vi "NXTMMX-DM.vi"(0 "Input of Motor Multiplexer":T4={"NXTMMX Address"=6, "Which Motor"=0, "Operation"=0, "Next Action"=0, "Position"=0, "Direction"=FALSE, "Power"=100, "Durartion"=0, "Wait for Completion"=FALSE, "Relative"=FALSE} {"Next Action" items=["Float", "Brake"]; "Operation" items=["Run Unlimited", "Run Seconds", "Run Tachometer"]; "Which Motor" items=["Motor 1", "Motor 2", "Both Motors"]; "NXTMMX Address" min=2 max=254 step=2 format="%x"}, 2 "NXT":T2={"error"={"status"=FALSE, "code"=0, "source"=""}, "address"="", "NXT #"=-1, "Show Error"=TRUE, "Connection"=4} {"Connection" items=["USB", "Bluetooth", "USB then Bluetooth", "Last Connection", "Preference"]}, 3 "Input Port":T3 items=["Port 1", "Port 2", "Port 3", "Port 4"]) -> (1 "Output of Motor Multiplexer":T1, 4 "NXT dup":T2={"error"={"status"=FALSE, "code"=0, "source"=""}, "address"="", "NXT #"=-1, "Show Error"=TRUE, "Connection"=4} {"Connection" items=["USB", "Bluetooth", "USB then Bluetooth", "Last Connection", "Preference"]})   [LabVIEW 2009]
uses:
  <vilib>/NXT/Block Support/NXT_InputPort.ctl
  <vilib>/NXT/Subs/LVHSConnector.ctl
  <vilib>/NXT/Block Support/HWPage.SensorType.ctl
  <vilib>/NXT/Block Support/HWPage.SensorMode.ctl
  <vilib>/NXT/Dual Mode Library/Waits/Wait_Num(msec).vi
panel:
  out "Address":i32
  # "mindsensors.com\nCopyright (c) 2009 by mindsensors.com\nEmail: info (<at>) mindsensors (<dot>) com\n\nThis program is free software. You can redistribute it and/or modify\nit under the terms of the GNU General Public License as published by\nthe Free Software Foundation; version 3 of the License.\nRead the license at: http://www.gnu.org/licenses/gpl.txt"
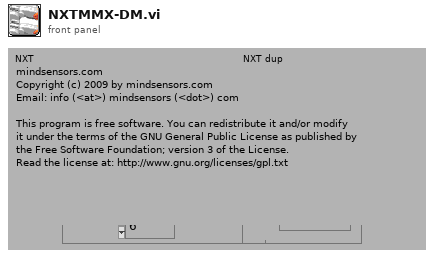
[diagram p1: front panel]
types:
  T1 = cluster{"Milivolts":u16, "Position 1":i32, "Position 2":i32, "Motor battery Voltage":dbl}
  T2 = typedef "LVHSConnector.ctl" = cluster{"error":errorcluster, "address":string, "NXT #":i32, "Show Error":bool, "Connection":u16}
  T3 = typedef "NXT_InputPort.ctl" = u8
  T4 = cluster{"NXTMMX Address":u8, "Which Motor":u8, "Operation":u8, "Next Action":u8, "Position":i32, "Direction":bool, "Power":i8, "Durartion":u8, "Wait for Completion":bool, "Relative":bool}
  T5 = typedef "HWPage.SensorType.ctl" = u8
  T6 = typedef "HWPage.SensorMode.ctl" = u8
  T7 = cluster{"millivolts":i16, "(hi.lo)":u16, "(hi.lo)":u16, dbl}
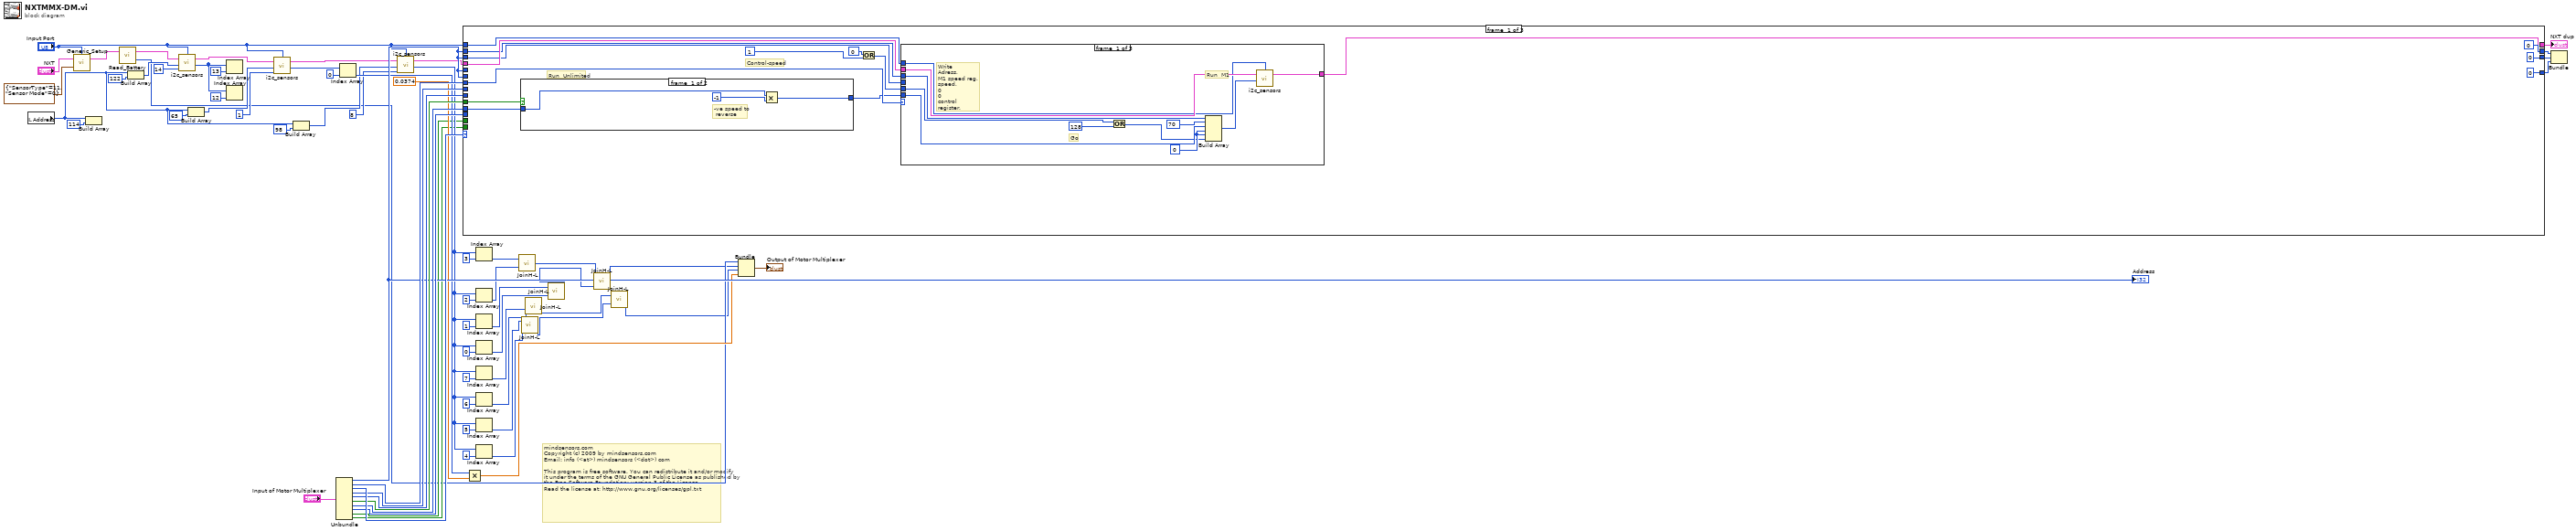
[diagram p0: block diagram]
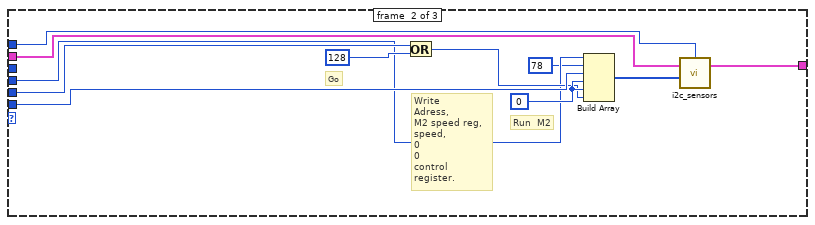
[diagram p2: hidden frame]
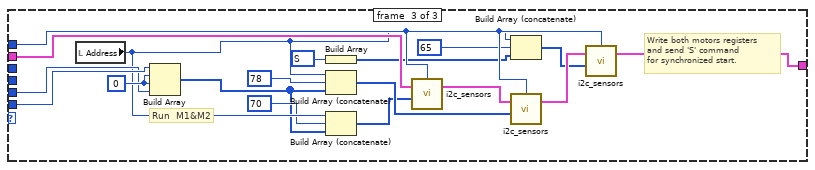
[diagram p3: hidden frame]
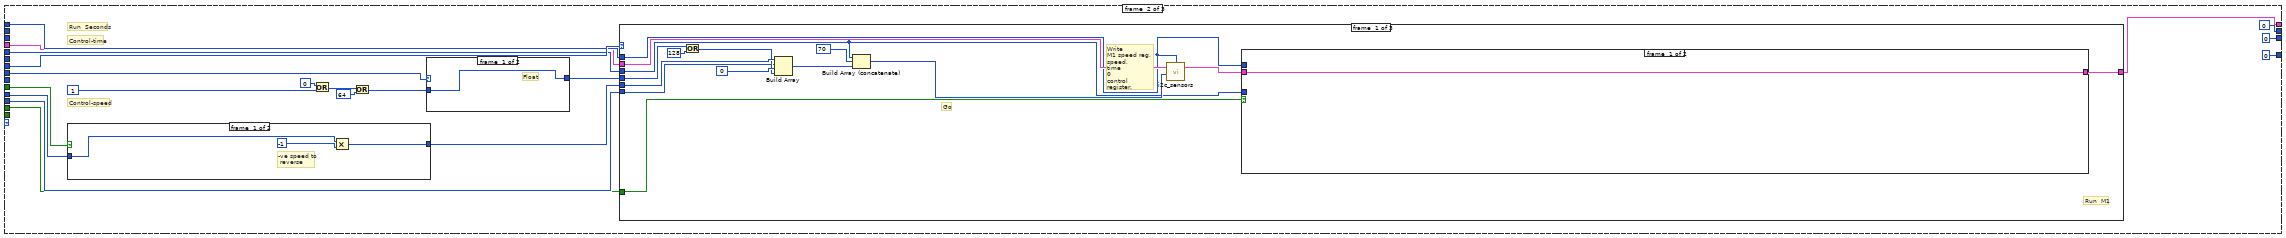
[diagram p5: hidden frame]
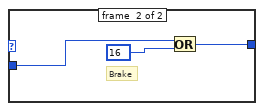
[diagram p6: hidden frame]
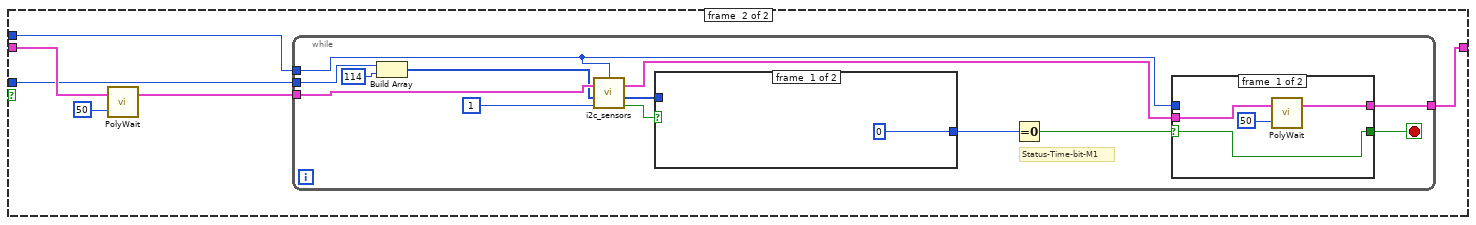
[diagram p7: hidden frame]
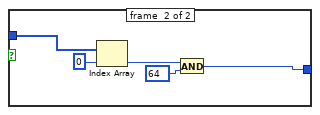
[diagram p9: hidden frame]
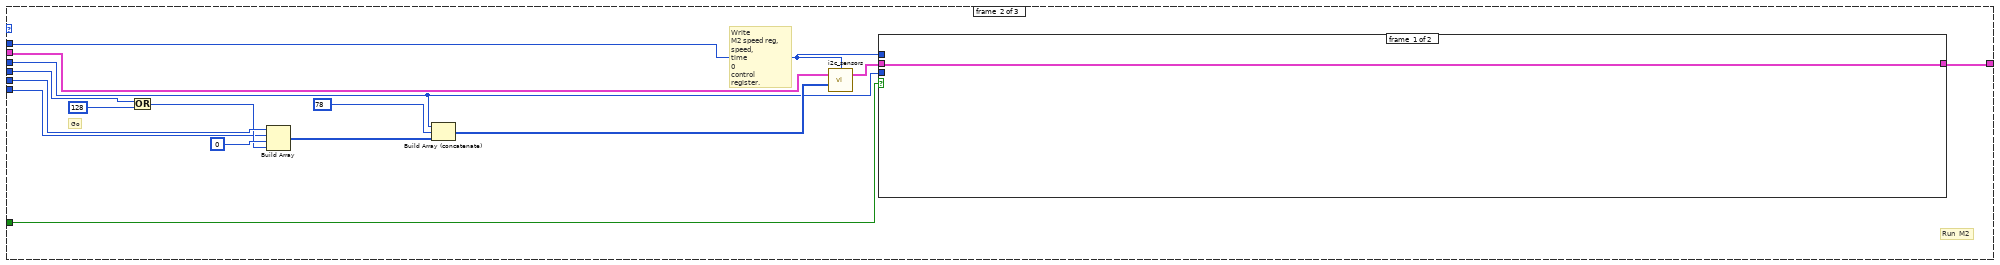
[diagram p10: hidden frame]
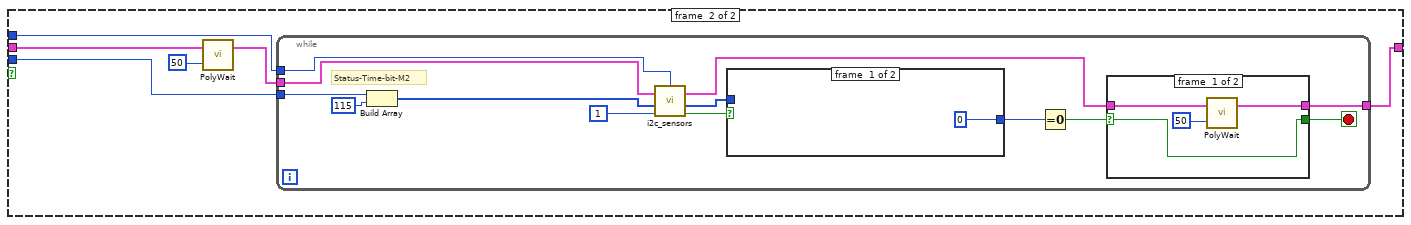
[diagram p11: hidden frame]
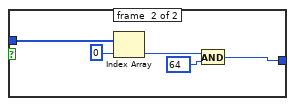
[diagram p13: hidden frame]
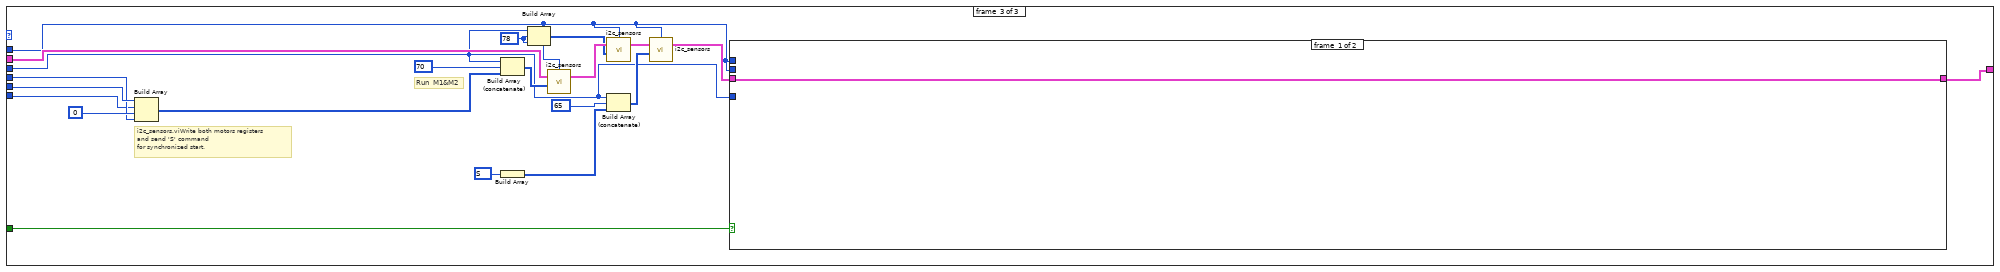
[diagram p14: hidden frame]
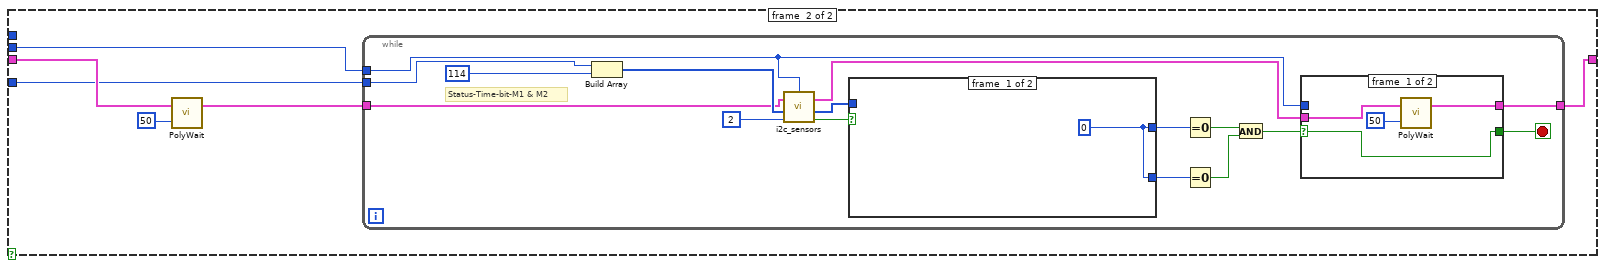
[diagram p15: hidden frame]
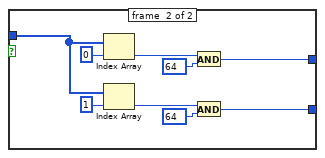
[diagram p17: hidden frame]
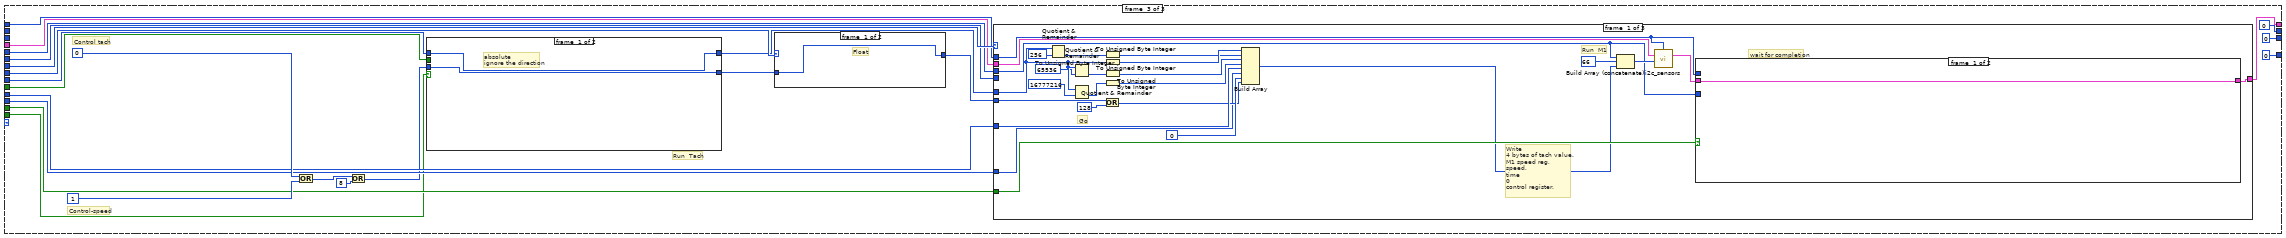
[diagram p19: hidden frame]
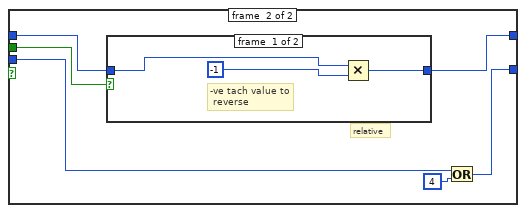
[diagram p20: hidden frame]
diagram:
  # "mindsensors.com\nCopyright (c) 2009 by mindsensors.com\nEmail: info (<at>) mindsensors (<dot>) com\n\nThis program is free software. You can redistribute it and/or modify\nit under the terms of the GNU General Public License as published by\nthe Free Software Foundation; version 3 of the License.\nRead the license at: http://www.gnu.org/licenses/gpl.txt"
  n1 = local read "Address"() -> (w25:i32)
  n2 = call <vilib>:"Generic_Setup.vi"("Sensor Setup"=cluster{"SensorType":T5, "Sensor Mode":T6} {"SensorType"=11, "Sensor Mode"=0}, "NXT"="NXT", "Port"="Input Port") -> ("NXT"=w57:T2)  [unwired: 1 out]
  n3 = Build Array(w25, u8 114 ("Reg Address")) -> ()  [unwired: 1 out]
  n4 = call <vilib>:"Read_Battery.vi"("NXT"=w57) -> ("millivolts"=w20:i16, "NXT"=w28:T2)  [unwired: 2 in]
  n5 = Build Array(w25, u8 122 ("Reg Address")) -> (w42:i32[])
  n6 = call <vilib>:"i2c_sensors.vi"("Return Length"=u8 14 ("bytes to read"), "Bytes to Write"=w42, "NXT"=w28, "Port"="Input Port") -> ("Bytes read"=w40:u8[], "NXT"=w35:T2)  [unwired: 1 in, 1 out]
  n7 = Build Array(w25, u8 65 ("Reg Address")) -> (w37:i32[])
  n8 = Index Array(array=w40, index=13) -> ()  [unwired: 1 out]
  n9 = Index Array(array=w40, index=12) -> ()  [unwired: 1 out]
  n10 = call <vilib>:"i2c_sensors.vi"("Return Length"=u8 1 ("bytes to read"), "Bytes to Write"=w37, "NXT"=w35, "Port"="Input Port") -> ("Bytes read"=w36:u8[], "NXT"=w30:T2)  [unwired: 1 in, 1 out]
  n11 = Build Array(w25, u8 98 ("Reg Address")) -> (w34:i32[])
  n12 = Unbundle("Input of Motor Multiplexer") -> ("NXTMMX Address"=w59:u8, "Which Motor"=w61:u8, "Operation"=w66:u8, "Next Action"=w65:u8, "Position"=w63:i32, "Direction"=w62:bool, "Power"=w64:i8, "Durartion"=w60:u8, "Wait for Completion"=w22:bool, "Relative"=w21:bool)
  "Address" <- w59
  n13 = Index Array(array=w36, index=0) -> (element=w45:u8)
  n14 = call <vilib>:"i2c_sensors.vi"("Return Length"=u8 8 ("bytes to read"), "Bytes to Write"=w34, "NXT"=w30, "Port"="Input Port") -> ("Bytes read"=w31:u8[], "NXT"=w26:T2)  [unwired: 1 in, 1 out]
  n15 = case shown="2" w66 {
    tunnel: w62 -> [w80 w144 w330]
    tunnel: w64 -> [w79 w143 w320]
    tunnel: w61 -> [w78 w142 w329]
    tunnel: "Input Port" -> [w76 w140 w328]
    tunnel: w60 -> [_ w137 w325]
    tunnel: w65 -> [_ w136 w324]
    tunnel: w63 -> [_ _ w321]
    tunnel: w22 -> [_ w133 w322]
    tunnel: w21 -> [_ _ w318]
    tunnel: [0 0 0] -> w19
    tunnel: [u32 0 ("Out") u32 0 ("Out") u32 0 ("Out")] -> w18
    tunnel: [u16 0 u16 0 u16 0] -> w17
    tunnel: w26 -> [w71 w129 w311]
    tunnel: [w70 w128 w312] -> w16
    tunnel: w59 -> [_ w127 w310]
    tunnel: w59 -> [w69 _ _]
    tunnel: w59 -> [_ _ w309]
    tunnel: w59 -> [w68 _ _]
    frame #0 {
      # "Control-speed"
      # "Run  Unlimited"
      n16 = case shown="False" w80 {
        tunnel: w79 -> [w125 w126]
        tunnel: [w123 w126] -> w77
        frame #0 {
          # "-ve speed to\n reverse"
          n17 = Multiply(x=w125, y=i8 -1) -> (x*y=w123:i8)
        }
        frame #1 {
        }
      }
      n18 = Or(x=0, y=1) -> (x .or. y?=w75:i32)
      n19 = case shown="2" w78 {
        tunnel: w75 -> [w92 w103 w119]
        tunnel: w77 -> [w91 w102 w122]
        tunnel: w76 -> [w86 w99 w114]
        tunnel: w71 -> [w88 w98 w118]
        tunnel: [w87 w97 w109] -> w70
        tunnel: w69 -> [w85 _ _]
        tunnel: w68 -> [_ w96 _]
        frame #0 {
          w90 = 0
          # "Go"
          # "Run  M1"
          # "Write \nAdress,\nM1 speed reg,\nspeed,\n0\n0\ncontrol register."
          n20 = Or(x=w92, y=128) -> (x .or. y?=w89:i32)
          n21 = Build Array(w85, 70, w91, w90, w90, w89) -> (w83:i32[])
          n22 = call <vilib>:"i2c_sensors.vi"("Bytes to Write"=w83, "NXT"=w88, "Port"=w86) -> ("NXT"=w87:T2)  [unwired: 2 in, 2 out]
        }
        frame #1 {
          w101 = 0
          # "Go"
          # "Run  M2"
          # "Write\nAdress, \nM2 speed reg,\nspeed,\n0\n0\ncontrol register."
          n23 = Or(x=w103, y=128) -> (x .or. y?=w100:i32)
          n24 = Build Array(w96, 78, w102, w101, w101, w100) -> (w94:i32[])
          n25 = call <vilib>:"i2c_sensors.vi"("Bytes to Write"=w94, "NXT"=w98, "Port"=w99) -> ("NXT"=w97:T2)  [unwired: 2 in, 2 out]
        }
        frame #2 {
          w120 = u16 83 items=["S"=83]
          w121 = 0
          # "Write both motors registers\nand send 'S' command \nfor synchronized start."
          # "Run  M1&M2"
          n26 = local read "Address"() -> (w108:i32)
          n27 = Build Array(w122, w121, w121, w119) -> (w105:i32[])
          n28 = Build Array(w120) -> (w112:u16[])
          n29 = Build Array (concatenate)(w108, 78, w105) -> (w116:i32[])
          n30 = Build Array (concatenate)(w108, 70, w105) -> (w106:i32[])
          n31 = call <vilib>:"i2c_sensors.vi"("Bytes to Write"=w106, "NXT"=w118, "Port"=w114) -> ("NXT"=w115:T2)  [unwired: 2 in, 2 out]
          n32 = Build Array (concatenate)(w108, 65, w112) -> (w110:i32[])
          n33 = call <vilib>:"i2c_sensors.vi"("Bytes to Write"=w116, "NXT"=w115, "Port"=w114) -> ("NXT"=w113:T2)  [unwired: 2 in, 2 out]
          n34 = call <vilib>:"i2c_sensors.vi"("Bytes to Write"=w110, "NXT"=w113, "Port"=w114) -> ("NXT"=w109:T2)  [unwired: 2 in, 2 out]
        }
      }
    }
    frame #1 {
      # "Control-time"
      # "Control-speed"
      # "Run  Seconds"
      n35 = case shown="False" w144 {
        tunnel: w143 -> [w307 w308]
        tunnel: [w305 w308] -> w141
        frame #0 {
          # "-ve speed to\n reverse"
          n36 = Multiply(x=w307, y=i8 -1) -> (x*y=w305:i8)
        }
        frame #1 {
        }
      }
      n37 = Or(x=0, y=1) -> (x .or. y?=w138:i32)
      n38 = Or(x=w138, y=64) -> (x .or. y?=w135:i32)
      n39 = case shown="0, Default" w136 {
        tunnel: w135 -> [w147 w149]
        tunnel: [w147 w150] -> w134
        frame #0 {
          # "Float"
        }
        frame #1 {
          # "Brake"
          n40 = Or(x=w149, y=16) -> (x .or. y?=w150:i32)
        }
      }
      n41 = case shown="2" w142 {
        tunnel: w134 -> [w164 w211 w262]
        tunnel: w141 -> [w163 w210 w265]
        tunnel: w140 -> [w153 w202 w247]
        tunnel: w137 -> [w160 w207 w261]
        tunnel: w133 -> [w159 w206 w260]
        tunnel: w129 -> [w157 w205 w256]
        tunnel: [w152 w199 w246] -> w128
        tunnel: w127 -> [w151 w198 w245]
        frame #0 {
          # "Go"
          # "Run  M1"
          # "Write \nM1 speed reg,\nspeed,\ntime\n0\ncontrol register."
          n42 = Or(x=w164, y=128) -> (x .or. y?=w161:i32)
          n43 = Build Array(w163, w160, 0, w161) -> (w154:i32[])
          n44 = Build Array (concatenate)(w151, 70, w154) -> (w156:i32[])
          n45 = call <vilib>:"i2c_sensors.vi"("Bytes to Write"=w156, "NXT"=w157, "Port"=w153) -> ("NXT"=w158:T2)  [unwired: 2 in, 2 out]
          n46 = case shown="True" w159 {
            tunnel: w153 -> [_ w172]
            tunnel: w158 -> [w166 w170]
            tunnel: [w166 w168] -> w152
            tunnel: w151 -> [_ w167]
            frame #0 {
            }
            frame #1 {
              n47 = call-poly <vilib>:"PolyWait.vi"("Time (100 msec)"=u16 50 ("Delay ms"), "NXT"=w170) -> ("NXT"=w169:T2)  [unwired: 2 in]
              n48 = while {
                tunnel: w172 -> [w176]
                tunnel: w169 -> [w181]
                tunnel: [w180] -> w168
                tunnel: w167 -> [w174]
                stop <- w184 stop-if-true
                # "Status-Time-bit-M1"
                n49 = Build Array(w174, 114) -> (w177:i32[])
                n50 = call <vilib>:"i2c_sensors.vi"("Return Length"=1, "Bytes to Write"=w177, "NXT"=w181, "Port"=w176) -> ("Success?"=w173:bool, "Bytes read"=w179:u8[], "NXT"=w182:T2)  [unwired: 1 in]
                n51 = case shown="True" w173 {
                  tunnel: w179 -> [_ w197]
                  tunnel: [u8 0 w193] -> w185
                  frame #0 {
                  }
                  frame #1 {
                    n52 = Index Array(array=w197, index=0) -> (element=w194:u8)
                    n53 = And(x=w194, y=u8 64) -> (x .and. y?=w193:u8)
                  }
                }
                n54 = Equal To 0?(x=w185) -> (x = 0?=w183:bool)
                n55 = case shown="False" w183 {
                  selector: w183 -> [w189 w191]
                  tunnel: w176 -> [_ _]
                  tunnel: [w189 w191] -> w184
                  tunnel: w182 -> [w187 w190]
                  tunnel: [w186 w190] -> w180
                  frame #0 {
                    n56 = call-poly <vilib>:"PolyWait.vi"("Time (100 msec)"=u16 50 ("Delay ms"), "NXT"=w187) -> ("NXT"=w186:T2)  [unwired: 2 in]
                  }
                  frame #1 {
                  }
                }
              }
            }
          }
        }
        frame #1 {
          # "Go"
          # "Run  M2"
          # "Write \nM2 speed reg,\nspeed,\ntime\n0\ncontrol register."
          n57 = Or(x=w211, y=128) -> (x .or. y?=w208:i32)
          n58 = Build Array(w210, w207, 0, w208) -> (w203:i32[])
          n59 = Build Array (concatenate)(w198, 78, w203) -> (w201:i32[])
          n60 = call <vilib>:"i2c_sensors.vi"("Bytes to Write"=w201, "NXT"=w205, "Port"=w202) -> ("NXT"=w200:T2)  [unwired: 2 in, 2 out]
          n61 = case shown="True" w206 {
            tunnel: w202 -> [_ w219]
            tunnel: w200 -> [w213 w217]
            tunnel: [w213 w215] -> w199
            tunnel: w198 -> [_ w214]
            frame #0 {
            }
            frame #1 {
              n62 = call-poly <vilib>:"PolyWait.vi"("Time (100 msec)"=u16 50 ("Delay ms"), "NXT"=w217) -> ("NXT"=w216:T2)  [unwired: 2 in]
              n63 = while {
                tunnel: w219 -> [w226]
                tunnel: w216 -> [w227]
                tunnel: [w229] -> w215
                tunnel: w214 -> [w221]
                stop <- w231 stop-if-true
                # "Status-Time-bit-M2"
                n64 = Build Array(w221, 115) -> (w223:i32[])
                n65 = call <vilib>:"i2c_sensors.vi"("Return Length"=1, "Bytes to Write"=w223, "NXT"=w227, "Port"=w226) -> ("Success?"=w220:bool, "Bytes read"=w222:u8[], "NXT"=w228:T2)  [unwired: 1 in]
                n66 = case shown="True" w220 {
                  tunnel: w222 -> [_ w244]
                  tunnel: [u8 0 w240] -> w232
                  frame #0 {
                  }
                  frame #1 {
                    n67 = Index Array(array=w244, index=0) -> (element=w241:u8)
                    n68 = And(x=w241, y=u8 64) -> (x .and. y?=w240:u8)
                  }
                }
                n69 = Equal To 0?(x=w232) -> (x = 0?=w230:bool)
                n70 = case shown="False" w230 {
                  selector: w230 -> [w236 w238]
                  tunnel: [w236 w238] -> w231
                  tunnel: [w234 w237] -> w229
                  tunnel: w228 -> [w233 w237]
                  frame #0 {
                    n71 = call-poly <vilib>:"PolyWait.vi"("Time (100 msec)"=u16 50 ("Delay ms"), "NXT"=w233) -> ("NXT"=w234:T2)  [unwired: 2 in]
                  }
                  frame #1 {
                  }
                }
              }
            }
          }
        }
        frame #2 {
          w263 = u16 83 items=["S"=83]
          w255 = 78
          # "i2c_sensors.viWrite both motors registers\nand send 'S' command \nfor synchronized start."
          # "Run  M1&M2"
          n72 = Build Array(w265, w261, 0, w262) -> (w258:i32[])
          n73 = Build Array (concatenate)(w245, 70, w258) -> (w257:i32[])
          n74 = Build Array(w263) -> (w253:u16[])
          n75 = Build Array(w245, w255, w255) -> (w250:i32[])
          n76 = call <vilib>:"i2c_sensors.vi"("Bytes to Write"=w257, "NXT"=w256, "Port"=w247) -> ("NXT"=w251:T2)  [unwired: 2 in, 2 out]
          n77 = call <vilib>:"i2c_sensors.vi"("Bytes to Write"=w250, "NXT"=w251, "Port"=w247) -> ("NXT"=w252:T2)  [unwired: 2 in, 2 out]
          n78 = Build Array (concatenate)(w245, 65, w253) -> (w249:i32[])
          n79 = call <vilib>:"i2c_sensors.vi"("Bytes to Write"=w249, "NXT"=w252, "Port"=w247) -> ("NXT"=w248:T2)  [unwired: 2 in, 2 out]
          n80 = case shown="True" w260 {
            tunnel: w247 -> [_ _]
            tunnel: w248 -> [w266 w271]
            tunnel: w247 -> [_ w269]
            tunnel: [w266 w268] -> w246
            tunnel: w245 -> [_ w267]
            frame #0 {
            }
            frame #1 {
              n81 = call-poly <vilib>:"PolyWait.vi"("Time (100 msec)"=u16 50 ("Delay ms"), "NXT"=w271) -> ("NXT"=w270:T2)  [unwired: 2 in]
              n82 = while {
                tunnel: w270 -> [w276]
                tunnel: w269 -> [w279]
                tunnel: [w275] -> w268
                tunnel: w267 -> [w274]
                stop <- w283 stop-if-true
                # "Status-Time-bit-M1 & M2"
                n83 = Build Array(w274, 114) -> (w280:i32[])
                n84 = call <vilib>:"i2c_sensors.vi"("Return Length"=2, "Bytes to Write"=w280, "NXT"=w276, "Port"=w279) -> ("Success?"=w273:bool, "Bytes read"=w278:u8[], "NXT"=w277:T2)  [unwired: 1 in]
                n85 = case shown="True" w273 {
                  tunnel: w278 -> [_ w303]
                  tunnel: [w295 w296] -> w288
                  tunnel: [w295 w298] -> w287
                  frame #0 {
                    w295 = u8 0
                  }
                  frame #1 {
                    n86 = Index Array(array=w303, index=0) -> (element=w299:u8)
                    n87 = Index Array(array=w303, index=1) -> (element=w297:u8)
                    n88 = And(x=w299, y=u8 64) -> (x .and. y?=w298:u8)
                    n89 = And(x=w297, y=u8 64) -> (x .and. y?=w296:u8)
                  }
                }
                n90 = Equal To 0?(x=w287) -> (x = 0?=w286:bool)
                n91 = Equal To 0?(x=w288) -> (x = 0?=w285:bool)
                n92 = And(x=w286, y=w285) -> (x .and. y?=w284:bool)
                n93 = case shown="True" w284 {
                  selector: w284 -> [w292 w294]
                  tunnel: w279 -> [_ _]
                  tunnel: [w292 w294] -> w283
                  tunnel: w277 -> [w290 w293]
                  tunnel: [w289 w293] -> w275
                  frame #0 {
                    n94 = call-poly <vilib>:"PolyWait.vi"("Time (100 msec)"=u16 50 ("Delay ms"), "NXT"=w290) -> ("NXT"=w289:T2)  [unwired: 2 in]
                  }
                  frame #1 {
                  }
                }
              }
            }
          }
        }
      }
    }
    frame #2 {
      # "Run  Tach"
      # "Control tach"
      # "Control-speed"
      n95 = Or(x=0, y=1) -> (x .or. y?=w326:i32)
      n96 = Or(x=w326, y=8) -> (x .or. y?=w317:i32)
      n97 = case shown="True" w318 {
        tunnel: w330 -> [_ w340]
        tunnel: w321 -> [w334 w339]
        tunnel: [w334 w338] -> w319
        tunnel: w317 -> [w333 w337]
        tunnel: [w333 w335] -> w316
        frame #0 {
          # "absolute\nignore the direction"
        }
        frame #1 {
          # "relative"
          n98 = case shown="False" w340 {
            tunnel: w339 -> [w343 w344]
            tunnel: [w341 w344] -> w338
            frame #0 {
              # "-ve tach value to\n reverse"
              n99 = Multiply(x=w343, y=i8 -1) -> (x*y=w341:i32)
            }
            frame #1 {
            }
          }
          n100 = Or(x=w337, y=4) -> (x .or. y?=w335:i32)
        }
      }
      n101 = case shown="0, Default" w324 {
        tunnel: [w345 w348] -> w323
        tunnel: w316 -> [w345 w346]
        frame #0 {
          # "Float"
        }
        frame #1 {
          # "Brake"
          n102 = Or(x=w346, y=16) -> (x .or. y?=w348:i32)
        }
      }
      n103 = case shown="0, Default" w329 {
        tunnel: w323 -> [w373 w431 w494]
        tunnel: w328 -> [w355 w412 w466]
        tunnel: w325 -> [w369 w427 w493]
        tunnel: w322 -> [w368 w426 w492]
        tunnel: w320 -> [w372 w430 w491]
        tunnel: w319 -> [w366 w419 w484]
        tunnel: [w349 w407 w479] -> w312
        tunnel: w311 -> [w352 w410 w478]
        tunnel: w310 -> [w350 _ _]
        tunnel: w309 -> [_ w408 _]
        frame #0 {
          # "wait for completion"
          # "Go"
          # "Run  M1"
          # "Write\n4 bytes of tach value. \nM1 speed reg,\nspeed,\ntime\n0\ncontrol register."
          n104 = Quotient & Remainder(x=w366, y=u32 256) -> (floor(x/y)=w362:u32)  [unwired: 1 out]
          n105 = Quotient & Remainder(x=w366, y=u32 65536) -> (floor(x/y)=w360:u32)  [unwired: 1 out]
          n106 = Quotient & Remainder(x=w366, y=u32 16777216) -> (floor(x/y)=w357:u32)  [unwired: 1 out]
          n107 = Or(x=w373, y=128) -> (x .or. y?=w370:i32)
          n108 = To Unsigned Byte Integer(number=w362) -> (unsigned 8bit integer=w361:u8)
          n109 = To Unsigned Byte Integer(number=w366) -> (unsigned 8bit integer=w367:u8)
          n110 = To Unsigned Byte Integer(number=w360) -> (unsigned 8bit integer=w359:u8)
          n111 = To Unsigned Byte Integer(number=w357) -> (unsigned 8bit integer=w358:u8)
          n112 = Build Array(w367, w361, w359, w358, w372, w369, 0, w370) -> (w356:i32[])
          n113 = Build Array (concatenate)(w350, 66, w356) -> (w353:i32[])
          n114 = call <vilib>:"i2c_sensors.vi"("Bytes to Write"=w353, "NXT"=w352, "Port"=w355) -> ("NXT"=w351:T2)  [unwired: 2 in, 2 out]
          n115 = case shown="True" w368 {
            tunnel: w355 -> [_ w381]
            tunnel: w351 -> [w375 w379]
            tunnel: w350 -> [_ w378]
            tunnel: [w375 w376] -> w349
            frame #0 {
            }
            frame #1 {
              n116 = call-poly <vilib>:"PolyWait.vi"("Time (100 msec)"=u16 50 ("Delay ms"), "NXT"=w379) -> ("NXT"=w377:T2)  [unwired: 2 in]
              n117 = while {
                tunnel: w381 -> [w389]
                tunnel: w378 -> [w387]
                tunnel: w377 -> [w386]
                tunnel: [w384] -> w376
                stop <- w392 stop-if-true
                # "Status-Tacho-bit-M1"
                n118 = Build Array(w387, 114) -> (w382:i32[])
                n119 = call <vilib>:"i2c_sensors.vi"("Return Length"=1, "Bytes to Write"=w382, "NXT"=w386, "Port"=w389) -> ("Success?"=w383:bool, "Bytes read"=w390:u8[], "NXT"=w385:T2)  [unwired: 1 in]
                n120 = case shown="True" w383 {
                  tunnel: w390 -> [_ w406]
                  tunnel: [u8 0 w402] -> w394
                  frame #0 {
                  }
                  frame #1 {
                    n121 = Index Array(array=w406, index=0) -> (element=w403:u8)
                    n122 = And(x=w403, y=u8 8) -> (x .and. y?=w402:u8)
                  }
                }
                n123 = Equal To 0?(x=w394) -> (x = 0?=w393:bool)
                n124 = case shown="True" w393 {
                  selector: w393 -> [w398 w400]
                  tunnel: w389 -> [_ _]
                  tunnel: [w398 w400] -> w392
                  tunnel: w385 -> [w396 w399]
                  tunnel: [w395 w399] -> w384
                  frame #0 {
                    n125 = call-poly <vilib>:"PolyWait.vi"("Time (100 msec)"=u16 50 ("Delay ms"), "NXT"=w396) -> ("NXT"=w395:T2)  [unwired: 2 in]
                  }
                  frame #1 {
                  }
                }
              }
            }
          }
        }
        frame #1 {
          # "Go"
          # "Run  M2"
          # "Write \nM2 speed reg,\nspeed,\ntime\n0\ncontrol register."
          n126 = Quotient & Remainder(x=w419, y=u32 256) -> (floor(x/y)=w422:u32)  [unwired: 1 out]
          n127 = Quotient & Remainder(x=w419, y=u32 65536) -> (floor(x/y)=w421:u32)  [unwired: 1 out]
          n128 = Quotient & Remainder(x=w419, y=u32 16777216) -> (floor(x/y)=w420:u32)  [unwired: 1 out]
          n129 = Or(x=w431, y=128) -> (x .or. y?=w428:i32)
          n130 = To Unsigned Byte Integer(number=w422) -> (unsigned 8bit integer=w417:u8)
          n131 = To Unsigned Byte Integer(number=w419) -> (unsigned 8bit integer=w418:u8)
          n132 = To Unsigned Byte Integer(number=w421) -> (unsigned 8bit integer=w416:u8)
          n133 = To Unsigned Byte Integer(number=w420) -> (unsigned 8bit integer=w415:u8)
          n134 = Build Array(w418, w417, w416, w415, w430, w427, 0, w428) -> (w413:i32[])
          n135 = Build Array (concatenate)(w408, 74, w413) -> (w411:i32[])
          n136 = call <vilib>:"i2c_sensors.vi"("Bytes to Write"=w411, "NXT"=w410, "Port"=w412) -> ("NXT"=w409:T2)  [unwired: 2 in, 2 out]
          n137 = case shown="True" w426 {
            tunnel: w412 -> [_ w439]
            tunnel: w409 -> [w433 w437]
            tunnel: w408 -> [_ w435]
            tunnel: [w433 w434] -> w407
            frame #0 {
            }
            frame #1 {
              n138 = call-poly <vilib>:"PolyWait.vi"("Time (100 msec)"=u16 50 ("Delay ms"), "NXT"=w437) -> ("NXT"=w436:T2)  [unwired: 2 in]
              n139 = while {
                tunnel: w439 -> [w443]
                tunnel: w436 -> [w449]
                tunnel: w435 -> [w447]
                tunnel: [w440] -> w434
                stop <- w450 stop-if-true
                # "Status-Tacho-bit-M2"
                n140 = Build Array(w447, 115) -> (w445:i32[])
                n141 = call <vilib>:"i2c_sensors.vi"("Return Length"=1, "Bytes to Write"=w445, "NXT"=w449, "Port"=w443) -> ("Success?"=w442:bool, "Bytes read"=w444:u8[], "NXT"=w441:T2)  [unwired: 1 in]
                n142 = case shown="True" w442 {
                  tunnel: w444 -> [_ w464]
                  tunnel: [u8 0 w460] -> w452
                  frame #0 {
                  }
                  frame #1 {
                    n143 = Index Array(array=w464, index=0) -> (element=w462:u8)
                    n144 = And(x=w462, y=u8 8) -> (x .and. y?=w460:u8)
                  }
                }
                n145 = Equal To 0?(x=w452) -> (x = 0?=w451:bool)
                n146 = case shown="True" w451 {
                  selector: w451 -> [w456 w458]
                  tunnel: w443 -> [_ _]
                  tunnel: [w456 w458] -> w450
                  tunnel: w441 -> [w454 w457]
                  tunnel: [w453 w457] -> w440
                  frame #0 {
                    n147 = call-poly <vilib>:"PolyWait.vi"("Time (100 msec)"=u16 50 ("Delay ms"), "NXT"=w454) -> ("NXT"=w453:T2)  [unwired: 2 in]
                  }
                  frame #1 {
                  }
                }
              }
            }
          }
        }
        frame #2 {
          w495 = u16 83 items=["S"=83]
          # "Write both motors registers\nand send 'S' command \nfor synchronized start."
          # "Run  M1&M2"
          n148 = Quotient & Remainder(x=w484, y=u32 256) -> (floor(x/y)=w487:u32)  [unwired: 1 out]
          n149 = Quotient & Remainder(x=w484, y=u32 65536) -> (floor(x/y)=w486:u32)  [unwired: 1 out]
          n150 = Quotient & Remainder(x=w484, y=u32 16777216) -> (floor(x/y)=w485:u32)  [unwired: 1 out]
          n151 = To Unsigned Byte Integer(number=w487) -> (unsigned 8bit integer=w482:u8)
          n152 = To Unsigned Byte Integer(number=w484) -> (unsigned 8bit integer=w483:u8)
          n153 = To Unsigned Byte Integer(number=w486) -> (unsigned 8bit integer=w481:u8)
          n154 = To Unsigned Byte Integer(number=w485) -> (unsigned 8bit integer=w480:u8)
          n155 = Build Array(w483, w482, w481, w480, w491, w493, 0, w494) -> (w469:i32[])
          n156 = local read "Address"() -> (w465:i32)
          n157 = Build Array (concatenate)(w465, 74, w469) -> (w474:i32[])
          n158 = Build Array (concatenate)(w465, 66, w469) -> (w472:i32[])
          n159 = Build Array(w495) -> (w467:u16[])
          n160 = call <vilib>:"i2c_sensors.vi"("Bytes to Write"=w472, "NXT"=w478, "Port"=w466) -> ("NXT"=w475:T2)  [unwired: 2 in, 2 out]
          n161 = call <vilib>:"i2c_sensors.vi"("Bytes to Write"=w474, "NXT"=w475, "Port"=w466) -> ("NXT"=w476:T2)  [unwired: 2 in, 2 out]
          n162 = Build Array (concatenate)(w465, 65, w467) -> (w473:i32[])
          n163 = call <vilib>:"i2c_sensors.vi"("Bytes to Write"=w473, "NXT"=w476, "Port"=w466) -> ("NXT"=w477:T2)  [unwired: 2 in, 2 out]
          n164 = case shown="True" w492 {
            tunnel: w466 -> [_ w503]
            tunnel: w477 -> [w497 w501]
            tunnel: [w497 w500] -> w479
            tunnel: w465 -> [_ w498]
            frame #0 {
            }
            frame #1 {
              n165 = call-poly <vilib>:"PolyWait.vi"("Time (100 msec)"=u16 50 ("Delay ms"), "NXT"=w501) -> ("NXT"=w499:T2)  [unwired: 2 in]
              n166 = while {
                tunnel: w503 -> [w508]
                tunnel: [w513] -> w500
                tunnel: w499 -> [w507]
                tunnel: w498 -> [w505]
                stop <- w514 stop-if-true
                # "Status-Tacho-bit-M1 & M2"
                n167 = Build Array(w505, 114) -> (w512:i32[])
                n168 = call <vilib>:"i2c_sensors.vi"("Return Length"=2, "Bytes to Write"=w512, "NXT"=w507, "Port"=w508) -> ("Success?"=w504:bool, "Bytes read"=w509:u8[], "NXT"=w506:T2)  [unwired: 1 in]
                n169 = case shown="True" w504 {
                  tunnel: w509 -> [_ w534]
                  tunnel: [w526 w527] -> w519
                  tunnel: [w526 w529] -> w518
                  frame #0 {
                    w526 = u8 0
                  }
                  frame #1 {
                    n170 = Index Array(array=w534, index=0) -> (element=w530:u8)
                    n171 = Index Array(array=w534, index=1) -> (element=w528:u8)
                    n172 = And(x=w530, y=u8 8) -> (x .and. y?=w529:u8)
                    n173 = And(x=w528, y=u8 8) -> (x .and. y?=w527:u8)
                  }
                }
                n174 = Equal To 0?(x=w518) -> (x = 0?=w517:bool)
                n175 = Equal To 0?(x=w519) -> (x = 0?=w516:bool)
                n176 = And(x=w517, y=w516) -> (x .and. y?=w515:bool)
                n177 = case shown="True" w515 {
                  selector: w515 -> [w523 w525]
                  tunnel: w508 -> [_ _]
                  tunnel: [w523 w525] -> w514
                  tunnel: [w521 w524] -> w513
                  tunnel: w506 -> [w520 w524]
                  frame #0 {
                    n178 = call-poly <vilib>:"PolyWait.vi"("Time (100 msec)"=u16 50 ("Delay ms"), "NXT"=w520) -> ("NXT"=w521:T2)  [unwired: 2 in]
                  }
                  frame #1 {
                  }
                }
              }
            }
          }
        }
      }
    }
  }
  "NXT dup" <- w16
  n179 = Multiply(x=w45, y=0.0374) -> (x*y=w24:dbl)
  n180 = Index Array(array=w31, index=3) -> (element=w14:u8)
  n181 = Index Array(array=w31, index=2) -> (element=w13:u8)
  n182 = Index Array(array=w31, index=1) -> (element=w12:u8)
  n183 = Index Array(array=w31, index=0) -> (element=w11:u8)
  n184 = Index Array(array=w31, index=7) -> (element=w10:u8)
  n185 = Index Array(array=w31, index=6) -> (element=w9:u8)
  n186 = Index Array(array=w31, index=5) -> (element=w8:u8)
  n187 = Index Array(array=w31, index=4) -> (element=w7:u8)
  n188 = call "JoinH-L.vi"("low"=w13, "hi"=w14) -> ("(hi.lo)"=w3:u16)
  n189 = call "JoinH-L.vi"("low"=w7, "hi"=w8) -> ("(hi.lo)"=w5:u16)
  n190 = call "JoinH-L.vi"("low"=w9, "hi"=w10) -> ("(hi.lo)"=w6:u16)
  n191 = call "JoinH-L.vi"("low"=w11, "hi"=w12) -> ("(hi.lo)"=w2:u16)
  n192 = call "JoinH-L.vi"("low"=w2, "hi"=w3) -> ("(hi.lo)"=w1:u16)
  n193 = call "JoinH-L.vi"("low"=w5, "hi"=w6) -> ("(hi.lo)"=w4:u16)
  n194 = Bundle("millivolts"=w20, "(hi.lo)"=w1, "(hi.lo)"=w4, w24) -> (→"Output of Motor Multiplexer":T7)  [unwired: 1 in]
  n195 = Bundle(w19, "Out"=w18, w17) -> ()  [unwired: 1 in, 1 out]
